vi "Get or Create Object Entry.vi"(8 "error in":errorcluster, 10 "OD Index":u16 format="%.0x", 11 "Obj Dict in":refnum<class "Object Dictionary.lvclass">) -> (0 "error out":errorcluster, 1 "Obj Entry":refnum<class "Object Entry.lvclass">, 3 "Obj Dict out":refnum<class "Object Dictionary.lvclass">)   [LabVIEW 2020, in "CANopen.lvlib" / "Object Dictionary.lvclass"]
uses:
  Object Dictionary.lvclass
  Object Dictionary.lvclass/Object Dictionary.ctl
  Object Entry/Object Entry.lvclass
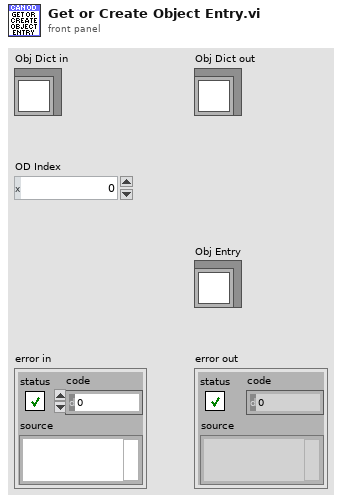
[diagram p1: front panel]
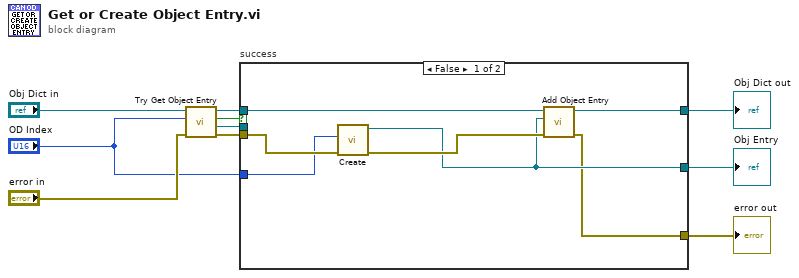
[diagram p0: block diagram]
diagram:
  n1 = call "Try Get Object Entry.vi"("error in"="error in", "Index"="OD Index", "Object Dictionary in"="Obj Dict in") -> ("error out"=w5:errorcluster, "Object Entry"=w1:refnum<class "Object Entry.lvclass">, "Success"=w2:bool, "Object Dictionary out"=w3:refnum<class "Object Dictionary.lvclass">)  [unwired: 5 in]
  n2 = case "success" shown="False" w2 {
    tunnel: w1 -> [_ w19]
    tunnel: w5 -> [w14 w20]
    tunnel: [w16 w19] -> w6
    tunnel: [w15 w20] -> w9
    tunnel: "OD Index" -> [w13 _]
    tunnel: [w12 w18] -> w4
    tunnel: w3 -> [w11 w18]
    frame False {
      n3 = call "Create.vi"("error in"=w14, "Index"=w13) -> ("error out"=w17:errorcluster, "Object Entry"=w16:refnum<class "Object Entry.lvclass">)  [unwired: 8 in]
      n4 = call "Add Object Entry.vi"("error in"=w17, "Obj Entry"=w16, "Obj Dict in"=w11) -> ("error out"=w15:errorcluster, "Obj Dict out"=w12:refnum<class "Object Dictionary.lvclass">)  [unwired: 7 in]
    }
    frame True {
    }
  }
  "error out" <- w9
  "Obj Dict out" <- w4
  "Obj Entry" <- w6
